vi "Read Command Core.vi"(8 "error in (no error)":errorcluster, 9 "timeout ms (5000)":i32=5000, 10 "Data":string, 11 "WSClient-P40001 in":refnum<class "WS Client.lvclass">) -> (0 "error out":errorcluster, 3 "WSClient-P40001 out":refnum<class "WS Client.lvclass">)   [LabVIEW 2016, in "WebSocket Networking.lvlib" / "WS Client.lvclass"]
doc: "--\nCopyright © 2017 Composed SystemsI All rights reserved.\n\nAuthor: Jon McBee <jon.mcbee@composed.io>\n\nThis library is provided \"AS IS\" ,WITHOUT WARRANTIES OR\nCONDITIONS OF ANY KIND, either express or implied.\n\nComposed Systems -- composed.io\n\nStream 0.0.1.1\nJon McBee - Composed Systems\nCopyright (c) 2017, Composed Systems"
uses:
  <userlib>/Common Components/WebSocket Networking/WS Client/WS Client.lvclass
  C:/Program Files (x86)/National Instruments/LabVIEW 2016/user.lib/Composed Systems/Stream/Mediator/Classes/Mediated Asynchronous Actor/Mediated Asynchronous Actor.lvclass
  <userlib>/Common Components/Common/command-data.ctl
  <userlib>/Common Components/Common/GUID-command-data.ctl
  <userlib>/Common Components/Common/Common.lvlib
  <userlib>/Composed Systems/Stream/Mediator/Classes/Mediated Asynchronous Actor/Mediated Asynchronous Actor.lvclass
  <userlib>/Common Components/WebSocket Networking/WS Server Msgs/WSserver Command Dispatch Msg/WSserver Command Dispatch Msg.lvclass
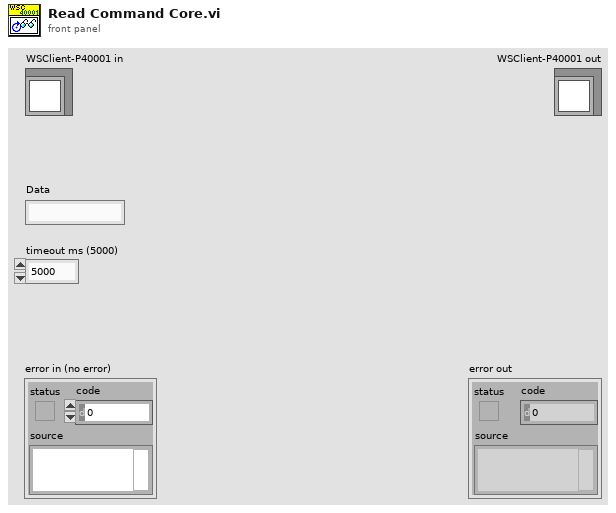
[diagram p1: front panel]
types:
  T1 = typedef "Common.lvlib/command-data.ctl" = cluster{"command":string, "data":string}
  T2 = typedef "Common.lvlib/GUID-command-data.ctl" = cluster{"GUID":string, "command":string, "data":string}
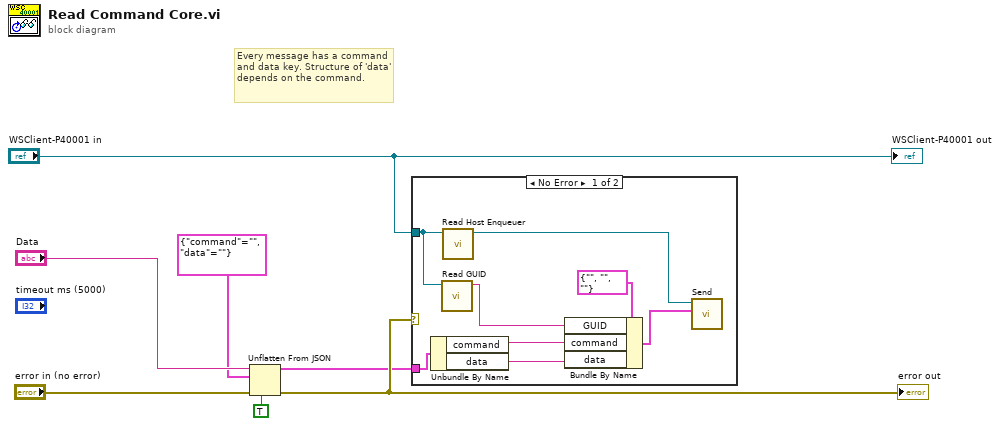
[diagram p0: block diagram]
diagram:
  # "Every message has a command and data key. Structure of 'data' depends on the command."
  n1 = Unflatten From JSON(JSON string="Data", type and defaults=T1 {"command"="", "data"=""}, default null elements? (F)=TRUE, error in (no error)="error in (no error)") -> (value=w1:T1, error out=w2:errorcluster)  [unwired: 3 in]
  "error out" <- w2
  n2 = case shown="No Error" w2 {
    tunnel: "WSClient-P40001 in" -> [w14 _]
    tunnel: w1 -> [w13 _]
    frame No Error {
      n3 = Unbundle By Name(w13) -> ("command"=w11:string, "data"=w10:string)
      n4 = call <userlib>:"Read GUID.vi"("Mediated Asynchronous Actor in"=w14) -> ("GUID"=w12:string)  [unwired: 10 in]
      n5 = call <userlib>:"Read Host Enqueuer.vi"("Mediated Asynchronous Actor in"=w14) -> ("Host Enqueuer"=w15:refnum<class "Message Transport Queue.lvclass">)  [unwired: 10 in]
      n6 = Bundle By Name(cluster=T2 {"GUID"="", "command"="", "data"=""} ("GUID-cmd-data"), "GUID"=w12, "command"=w11, "data"=w10) -> (w8:T2)
      n7 = call <userlib>:"Send.vi"("GUID-cmd-data"=w8, "Message Transport Queue"=w15) -> ()  [unwired: 9 in, 1 out]
    }
    frame Error {
    }
  }
  "WSClient-P40001 out" <- "WSClient-P40001 in"
